vi "Log File.vi"(0 "Version":string, 1 "ID":string, 3 "Checksums":string[](array[string]), 5 "Java":string, 7 "URL":string, 9 "DataProcessor.exe?":string, 11 "error in":errorcluster, 12 "Pass?":string, 14 "Error":string) -> (4 "File Name":string, 15 "error out":errorcluster)   [LabVIEW 2021]
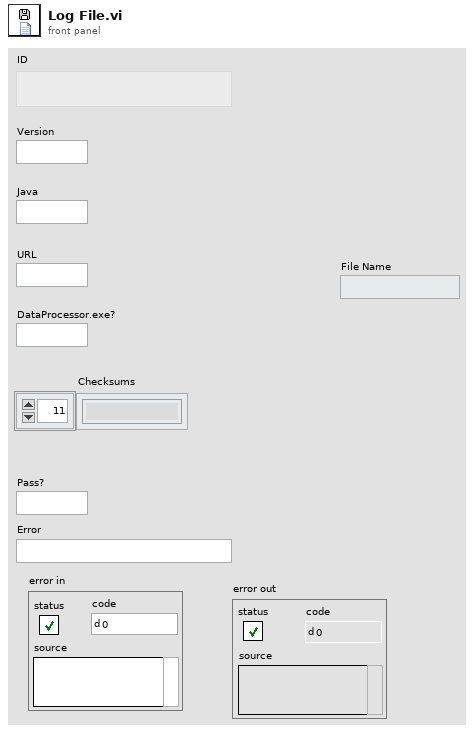
[diagram p1: front panel]
types:
  T1 = enum16{"open", "replace", "create", "open or create", "replace or create", "replace or create with confirmation"}
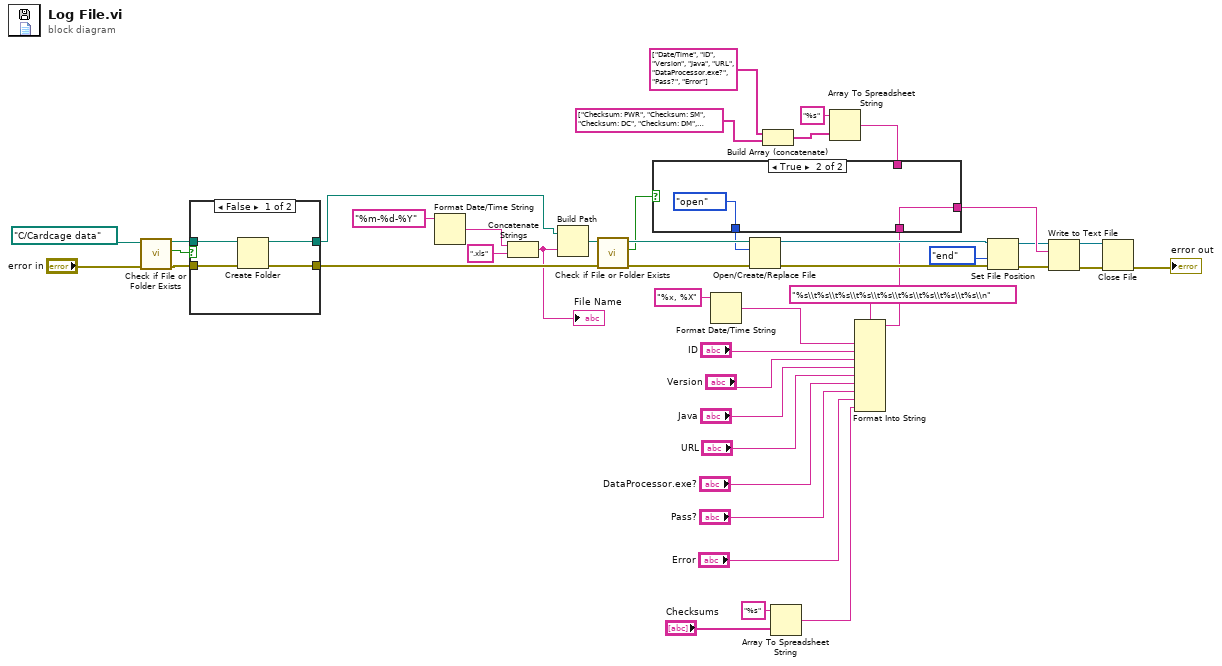
[diagram p0: block diagram]
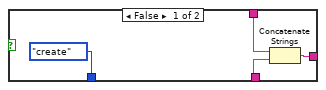
[diagram p3: hidden frame]
diagram:
  n1 = call <vilib>:"Check if File or Folder Exists.vi"("error in (no error)"="error in", "path"=path "C:/Cardcage data") -> ("error out"=w15:errorcluster, "file or folder exists?"=w17:bool, "dup path"=w16:path)  [unwired: 7 in]
  n2 = case shown="False" w17 {
    tunnel: w16 -> [w48 w50]
    tunnel: w15 -> [w47 w49]
    tunnel: [w46 w50] -> w13
    tunnel: [w45 w49] -> w14
    frame False {
      n3 = Create Folder(path (use dialog)=w48, error in=w47) -> (created path=w46:path, error out=w45:errorcluster)  [unwired: 1 in, 1 out]
    }
    frame True {
    }
  }
  n4 = Format Date/Time String(time format string (%c)="%m-%d-%Y") -> (date/time string=w20:string)  [unwired: 2 in]
  n5 = Concatenate Strings(w20, ".xls" ("time format string (%c)")) -> (w1:string)
  "File Name" <- w1
  n6 = Build Path(base path=w13, name or relative path=w1) -> (appended path=w26:path)
  n7 = call <vilib>:"Check if File or Folder Exists.vi"("error in (no error)"=w14, "path"=w26) -> ("error out"=w34:errorcluster, "file or folder exists?"=w30:bool, "dup path"=w33:path)  [unwired: 7 in]
  n8 = Format Date/Time String(time format string (%c)="%x, %X") -> (date/time string=w23:string)  [unwired: 2 in]
  n9 = Build Array (concatenate)(string[] ["Date/Time", "ID", "Version", "Java", "URL", "DataProcessor.exe?", "Pass?", "Error"], string[] ["Checksum: PWR", "Checksum: SM", "Checksum: DC", "Checksum: DM", "Checksum: WS", "Checksum: DS", "Checksum: WC", "Checksum: WA", "Checksum: WM", "Checksum: DA", "Checksum: WH", "Checksum: DH"] ("Array")) -> (w6:string[])
  n10 = Array To Spreadsheet String(array="Checksums", 3:"%s" ("format string")) -> (spreadsheet string=w2:string)  [unwired: 1 in]
  n11 = Array To Spreadsheet String(array=w6, 3:"%s" ("format string")) -> (spreadsheet string=w41:string)  [unwired: 1 in]
  n12 = Format Into String(format string="%s\\t%s\\t%s\\t%s\\t%s\\t%s\\t%s\\t%s\\t%s\\n", w23, "ID", "Version", "Java", "URL", "DataProcessor.exe?", "Pass?", "Error", w2) -> (resulting string=w27:string)  [unwired: 2 in, 1 out]
  n13 = case shown="True" w30 {
    tunnel: w41 -> [w54 _]
    tunnel: [w53 w55] -> w40
    tunnel: [T1."create" ("operation (0:open)") T1."open" ("operation (0:open)")] -> w29
    tunnel: w27 -> [w51 w55]
    frame False {
      n14 = Concatenate Strings(w54, w51) -> (w53:string)
    }
    frame True {
    }
  }
  n15 = Open/Create/Replace File(file path (use dialog)=w33, error in=w34, operation (0:open)=w29) -> (refnum out=w32:refnum<file>, error out=w31:errorcluster)  [unwired: 3 in, 1 out]
  n16 = Set File Position(refnum=w32, from (0:start)=enum16{"start", "end", "current"}."end", error in=w31) -> (refnum out=w37:refnum<file>, error out=w36:errorcluster)  [unwired: 1 in]
  n17 = Write to Text File(file (use dialog)=w37, text=w40, error in=w36) -> (refnum out=w38:refnum<file>, error out=w39:errorcluster)  [unwired: 1 in, 1 out]
  n18 = Close File(refnum=w38, error in=w39) -> (error out=→"error out":errorcluster)  [unwired: 1 out]
